vi "Accelerometer 3D.vi"() -> ()   [LabVIEW 2025]
panel:
  in  "Pin_Z":u8=36
  in  "Pin_Y":u8=39
  in  "Pin_X":u8=34
  in  "Calibrar":bool
  out "3D Picture":refnum<vi>(3d-picture)
  out "Z":u16
  out "Y":u16
  out "X":u16
  in  "VISA resource name":refnum<visa-resource-name>
  out "error out":errorcluster
  in  "stop":bool
  in  "Color":u32(colorbox)
  # "Ejemplo: Uso de acelerómetro analógico (ADXL335)\nEste ejemplo muestra cómo adquirir y visualizar las señales de un acelerómetro analógico tipo ADXL335 en LV_ESP32, incluyendo la representación gráfica de las rotaciones"
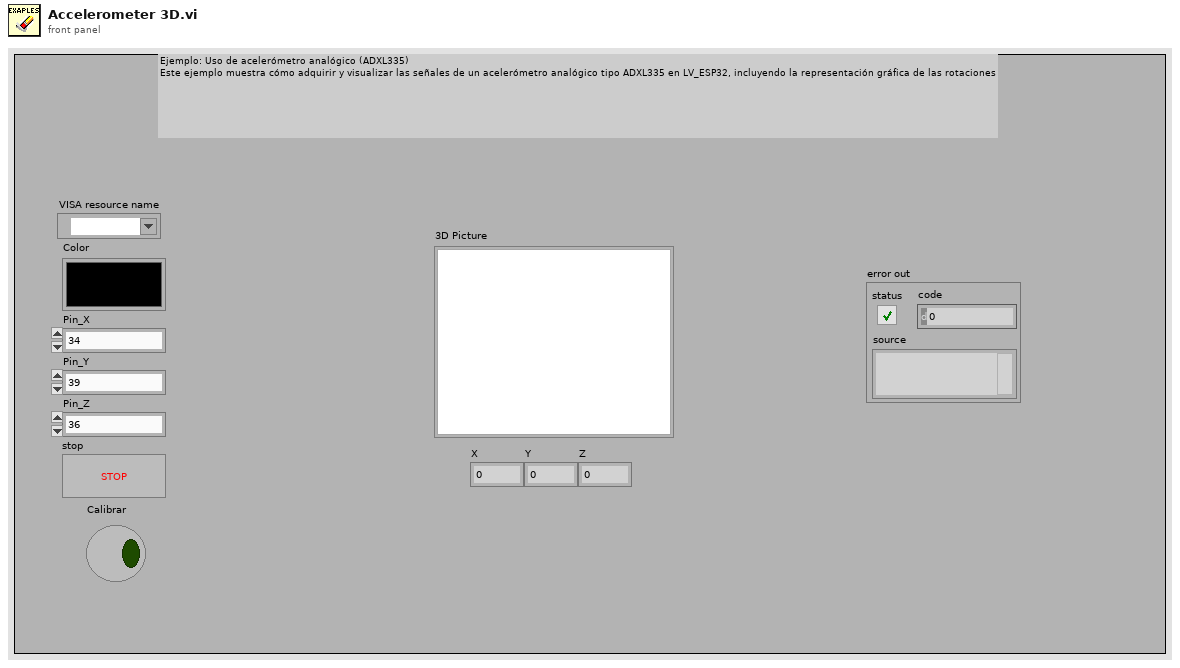
[diagram p1: front panel]
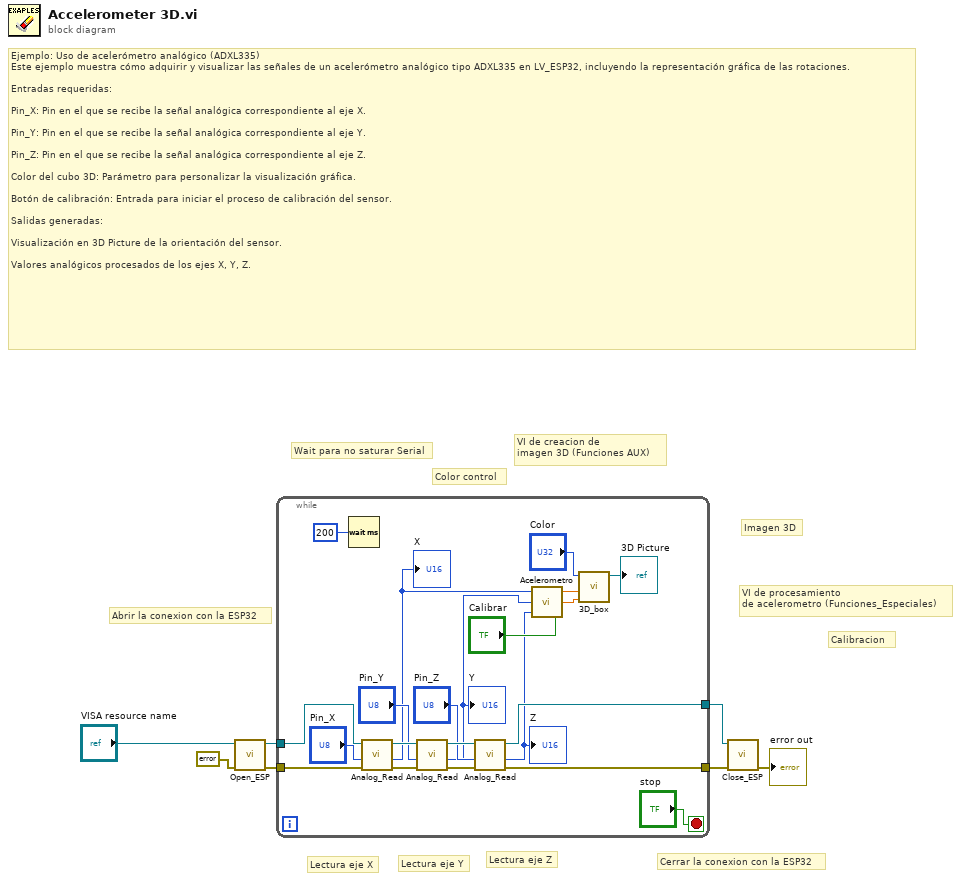
[diagram p0: block diagram]
diagram:
  # "Color control"
  # "Imagen 3D"
  # "VI de creacion de \nimagen 3D (Funciones AUX)"
  # "VI de procesamiento \nde acelerometro (Funciones_Especiales)"
  # "Calibracion"
  # "Cerrar la conexion con la ESP32"
  # "Lectura eje Z"
  # "Lectura eje Y"
  # "Lectura eje X"
  # "Wait para no saturar Serial"
  # "Abrir la conexion con la ESP32"
  # "Ejemplo: Uso de acelerómetro analógico (ADXL335)\nEste ejemplo muestra cómo adquirir y visualizar las señales de un acelerómetro analógico tipo ADXL335 en LV_ESP32, incluyendo la representación gráfica de las rotaciones.\n\nEntradas requeridas:\n\nPin_X: Pin en el que se recibe la señal analógica correspondiente al eje X.\n\nPin_Y: Pin en el que se recibe la señal analógica correspondiente al eje Y.\n\nPin_Z: Pin en el que se recibe la señal analógica correspondiente al eje Z.\n\nColor del cubo 3D: Parámetro para personalizar la visualización gráfica.\n\nBotón de calibración: Entrada para iniciar el proceso de calibración del sensor.\n\nSalidas generadas:\n\nVisualización en 3D Picture de la orientación del sensor.\n\nValores analógicos procesados de los ejes X, Y, Z."
  n1 = call "Open_ESP.vi"("error in (no error)"=errorcluster {"status"=FALSE, "code"=0, "source"=""}, "VISA resource name"="VISA resource name") -> ("error out"=w6:errorcluster, "VISA resource name out"=w5:refnum<visa-resource-name>)  [unwired: 8 in]
  n2 = while {
    tunnel: [w24] -> w7
    tunnel: w6 -> [w22]
    tunnel: w5 -> [w21]
    tunnel: [w16] -> w4
    stop <- "stop" stop-if-true
    n3 = Wait (ms)(milliseconds to wait=u32 200) -> ()  [unwired: 1 out]
    n4 = call "Analog_Read.vi"("error in (no error)"=w22, "Pin"="Pin_X", "VISA resource name"=w21) -> ("error out"=w23:errorcluster, "Analog read"=w8:u16, "VISA resource name out"=w20:refnum<visa-resource-name>)  [unwired: 6 in]
    "X" <- w8
    n5 = call "Analog_Read.vi"("error in (no error)"=w23, "Pin"="Pin_Y", "VISA resource name"=w20) -> ("error out"=w26:errorcluster, "Analog read"=w9:u16, "VISA resource name out"=w25:refnum<visa-resource-name>)  [unwired: 6 in]
    "Y" <- w9
    n6 = call "Analog_Read.vi"("error in (no error)"=w26, "Pin"="Pin_Z", "VISA resource name"=w25) -> ("error out"=w24:errorcluster, "Analog read"=w10:u16, "VISA resource name out"=w16:refnum<visa-resource-name>)  [unwired: 6 in]
    "Z" <- w10
    n7 = call "Acelerometro.vi"("Calibrar"="Calibrar", "Analog read Z"=w10, "Analog read Y"=w9, "Analog read X"=w8) -> ("PITCH"=w12:dbl, "ROLL"=w13:dbl)
    n8 = call "3D_box.vi"("PITCH"=w12, "ROLL"=w13, "Color"="Color") -> ("3D Picture"=→"3D Picture":refnum<vi>)  [unwired: 8 in]
  }
  n9 = call "Close_ESP.vi"("error in (no error)"=w7, "VISA resource name"=w4) -> ("error out"=→"error out":errorcluster)  [unwired: 9 in]
